vi "Forebrain Draw Buoy.vi"() -> ()   [LabVIEW 2012]
doc: "This VI contrains the Forebrain within the Olin Robot Architecture. It must be run first to load the appropriate mission definition files. It contains a finite state machine built around a tabbed Operator interface that will guide an operator through the startup, run shutdown mission sequence. After running it, run the Midbrain and Hindbrain VIS."
panel:
  in  "# 5":u8 max=5 step=1
  in  "# 4":u8 max=5 step=1
  in  "# 3":u8 max=5 step=1
  in  "# 2":u8 max=5 step=1
  in  "# 1":u8 max=5 step=1
  in  "# 0":u8 max=5 step=1
  in  "IR Servo":u8(knob)=7 scale=0.0..14.0
  out "return count":u32
  out "error out":errorcluster
  in  "error in 2":errorcluster
  out "Desired \nVelocity":i16=5
  out "Local\nHeading":i16=90
  out "Ycurrent":dbl format="%#_3g"
  out "Xcurrent":dbl format="%#_3g"
  out "Ystart":dbl
  out "Xstart":dbl
  in  "error in":errorcluster
  out "Robot Live":bool
  in  "E-Stop":bool
  in  "Tab":T1(tab)
  out "MissionTime (Min)":dbl(knob) scale=0.0..10.0
  out "LidarDist":i16
  out "IR Index":i32
  out "BatteryLevel":dbl(slide) scale=6.0..9.0
  out "String Received":string
  out "Send String":string="$B^"
  in  "VISA resource name":refnum<visa-resource-name>="COM10"
  in  "Mode":i16 min=0 max=99 step=1
  in  "Desired Vel":i16(slide) scale=-9.0..9.0
  in  "Local Head":i16(slide) scale=-180.0..180.0
  out "StartMissionMap":picture
  out "MapDARCheck":picture
  in  "RunRobot":bool
  in  "Tug letter":string="G"
  out "Tug X":i32
  out "Tug Y":i32
  out "Tug H":i32
  out "BS Time Out?":bool
  out "Buoy locations":cluster{"regular expression":string, i32, i32}[](array[cluster])
  out "Valid ?":bool
  out "Battery\nVolts":i16
  out "Base Station data rec'd":string
  out "udp rate":bool
  out "CollisionWarning":bool
  out "DebugMapDAR":picture
  in  "MapDAR Control":T2={"NumberOfBeams"=180, "SensorRange"=500.0, "Noise (0.1 to 1)"=0.0} {"Noise (0.1 to 1)" min=0.0 max=1.0 step=0.1; "SensorRange" min=500.0 max=1500.0 step=100.0; "NumberOfBeams" min=36 max=360 step=2}
  out "MapDAR Data (r:pixel b:degrees)":cluster{"Range":dbl, "Bearing":dbl}[](array[cluster])
  in  "Stop DebugSENSE":bool
  out "MissionMap":picture
  out "Tug position":T3
  out "initialized MDF":T4(array[cluster])
  out "Way Point Index":i32
  out "InitialWaypoint":cluster{"X":i16, "Y":i16}
  in  "Pen Color":u32(colorbox)=15671808
  in  "Select Pen Attributes":T5={"Width"=1, "Style"=enum."Solid"}
  out "Draw??":bool
  in  "WhereAmI?FromBase":T6
  out "(xr,yr)":cluster{"X":dbl, "Y":dbl}
  in  "RobotPosition":T3 {"xrobot" min=0.0 max=1177.0 step=10.0; "yrobot" min=0.0 max=850.0 step=10.0; "heading" min=0.0 max=7.0 step=0.1}
  out "MDF_Original":T4(array[cluster])
  out "WhatAroundMeMap?":cluster{"T":dbl, "Range":dbl, "Bearing":dbl}[](array[cluster])
  out "WayPointAct":dbl[](array[numeric])
  out "SteerAngle":dbl
  out "MissionDefFile":picture
  out "MDF":T4(array[cluster])
  in  "Select Your Behavior":T7(ring)
  out "No. of Waypoints":i32
  in  "Exit Planning":bool
  in  "BoatSpeed for Leg":dbl(slide) min=-9.0 max=9.0 step=1.0 scale=-9.0..9.0
  out "BuildMDF":bool
  out "WayPoint Position":cluster{"X":i32, "Y":i32}
  out "Send String to NXT":string="$B^"
  in  "Behavior Command":T7(ring)
  out "CollisionLight":bool
  out "Where? Manual":T6
  out "ActManual":bool
  in  "Manual Heading":i16(knob) min=-179 max=180 step=5 scale=180.0..-180.0
  out "MWhat?":bool
  out "Where? 2":bool
  out "How? 2":bool
  in  "ManualModeStop":bool
  out "ManualModeMapDAR":picture
  out "ManualMissionMap":picture
  out "Battery":dbl(slide) scale=0.0..8.0
  in  "Manual Vel":dbl(slide) min=-6.0 max=6.0 step=1.0 scale=-6.0..6.0
  out "MissionTime":dbl(knob) scale=0.0..10.0
  out "Heading":cluster{dbl, dbl}(knob)={0.0, 34.390870865624734} scale=180.0..-179.0 scale format="%#_3g"
  out "Speed":i16(knob) scale=-6.0..6.0
  out "Current Behavior":T7(ring)
  out "Robot Position":cluster{"X":dbl, "Y":dbl} {"X" format="%#_3g"; "Y" format="%#_3g"}
  out "Ready":bool
  in  "Pause":bool
  in  "Rerun MDF":bool
  out "CollisionLight 2":bool
  out "Act":bool
  out "Neo-C":bool
  out "How?":bool
  out "What?":bool
  out "A Heading":cluster{dbl, dbl}(knob)={0.0, 34.390870865624734} scale=180.0..-180.0
  out "A Speed":dbl(knob) scale=-9.0..9.0
  out "AutoBattery":dbl(slide) scale=0.0..8.0
  out "AutoModeLIDAR":picture
  out "AutoMissionMap":picture
  in  "RunAutoMode":bool
  out "MissionTimeAuto":dbl(knob) scale=0.0..60.0
  out "Where?":bool
  # "To run\nrobot,\nclick\narrow\nabove\n\nRun Robot button must be on"
  # "Operation Directions\n\n1)Click on Startup&\nShutdown tab.\n2) Click on Run \nArrow on menubar.\nRun Forebrain,\nvis from the project\nexplorer.\n3) Select a mssion \nmap file when asked.\n4) Check robot is \nfully operational on\nStartup tab.\n5) Debug with debug\ntabs as required.\n6) Select ManualMode\ntab and test drive \nrobot.\n7) Select PlanMission\ntab and set up \nmission.\n8) Go to AutoMode\ntab and run mission."
  # "Turns off drive\nmotors"
  # "Enter Olin Test  Pool"
  # "Xbee Com Port"
  # "xBee\"Send String\" (mode, desired velocity, local heading)"
  # "(Type in Tug Letter  L T G P  (look at boat cradle)"
  # "Should be on to\nrun"
  # "BoatG,X,Y,H,BoatT,X,Y,H,BoatP,X,Y.H,BoatL,X,Y,H,BuoyA,X,Y,BuoyB,X,Y,BuoyC,X,Y,BuoyD,X,Y,Time(hours,Min,Sec)"
  # "To stop  program \nturn off here"
  # "Use this tab\nto explore\nLIDAR\ndata and \noperation"
  # "Set\nNumberOfBeams\nSensorRange\nNoise\nto\nview\nsimulated\nsensor\ndata"
  # "Turn Debug Sim \nto leave this\ntab--->"
  # "This tab will auto\nreturn to Startup \nin 2 seconds"
  # "Clean up interface and make more useful for debugging behaviors"
  # "Build out interface and make more useful for debugging act"
  # "This tab will auto\nreturn to Startup \nin 2 seconds"
  # "Directions:\n1) Select Robot Behavior for each mission leg.\n2) Select Robot Speed for leg.\n3) Click on robots current location for first waypoint.\n4) Hold down button and drag to next\nwaypoint. Click on next leg waypoint.\n5) Hold mouse button down and drag to \nnext waypoint. \n6) Click on next waypoint. Repeat for full mission.\n7) MDF will store up to 20 waypoints."
  # "Remember to\nset boat\nleg speed !"
  # "Please Adjust Scroll Barrs in Tug Off Mode to Prevent  Extra Lines Being Drawn"
  # "\"Send String\" (mode, desired velocity, local heading)"
  # "Press to stop and return to StartUp"
  # "Open MidBrain\nArbiter to see\nBrain Waves"
  # "AutoMode\nAutomatically \nReturns to \nStartUp Mode"
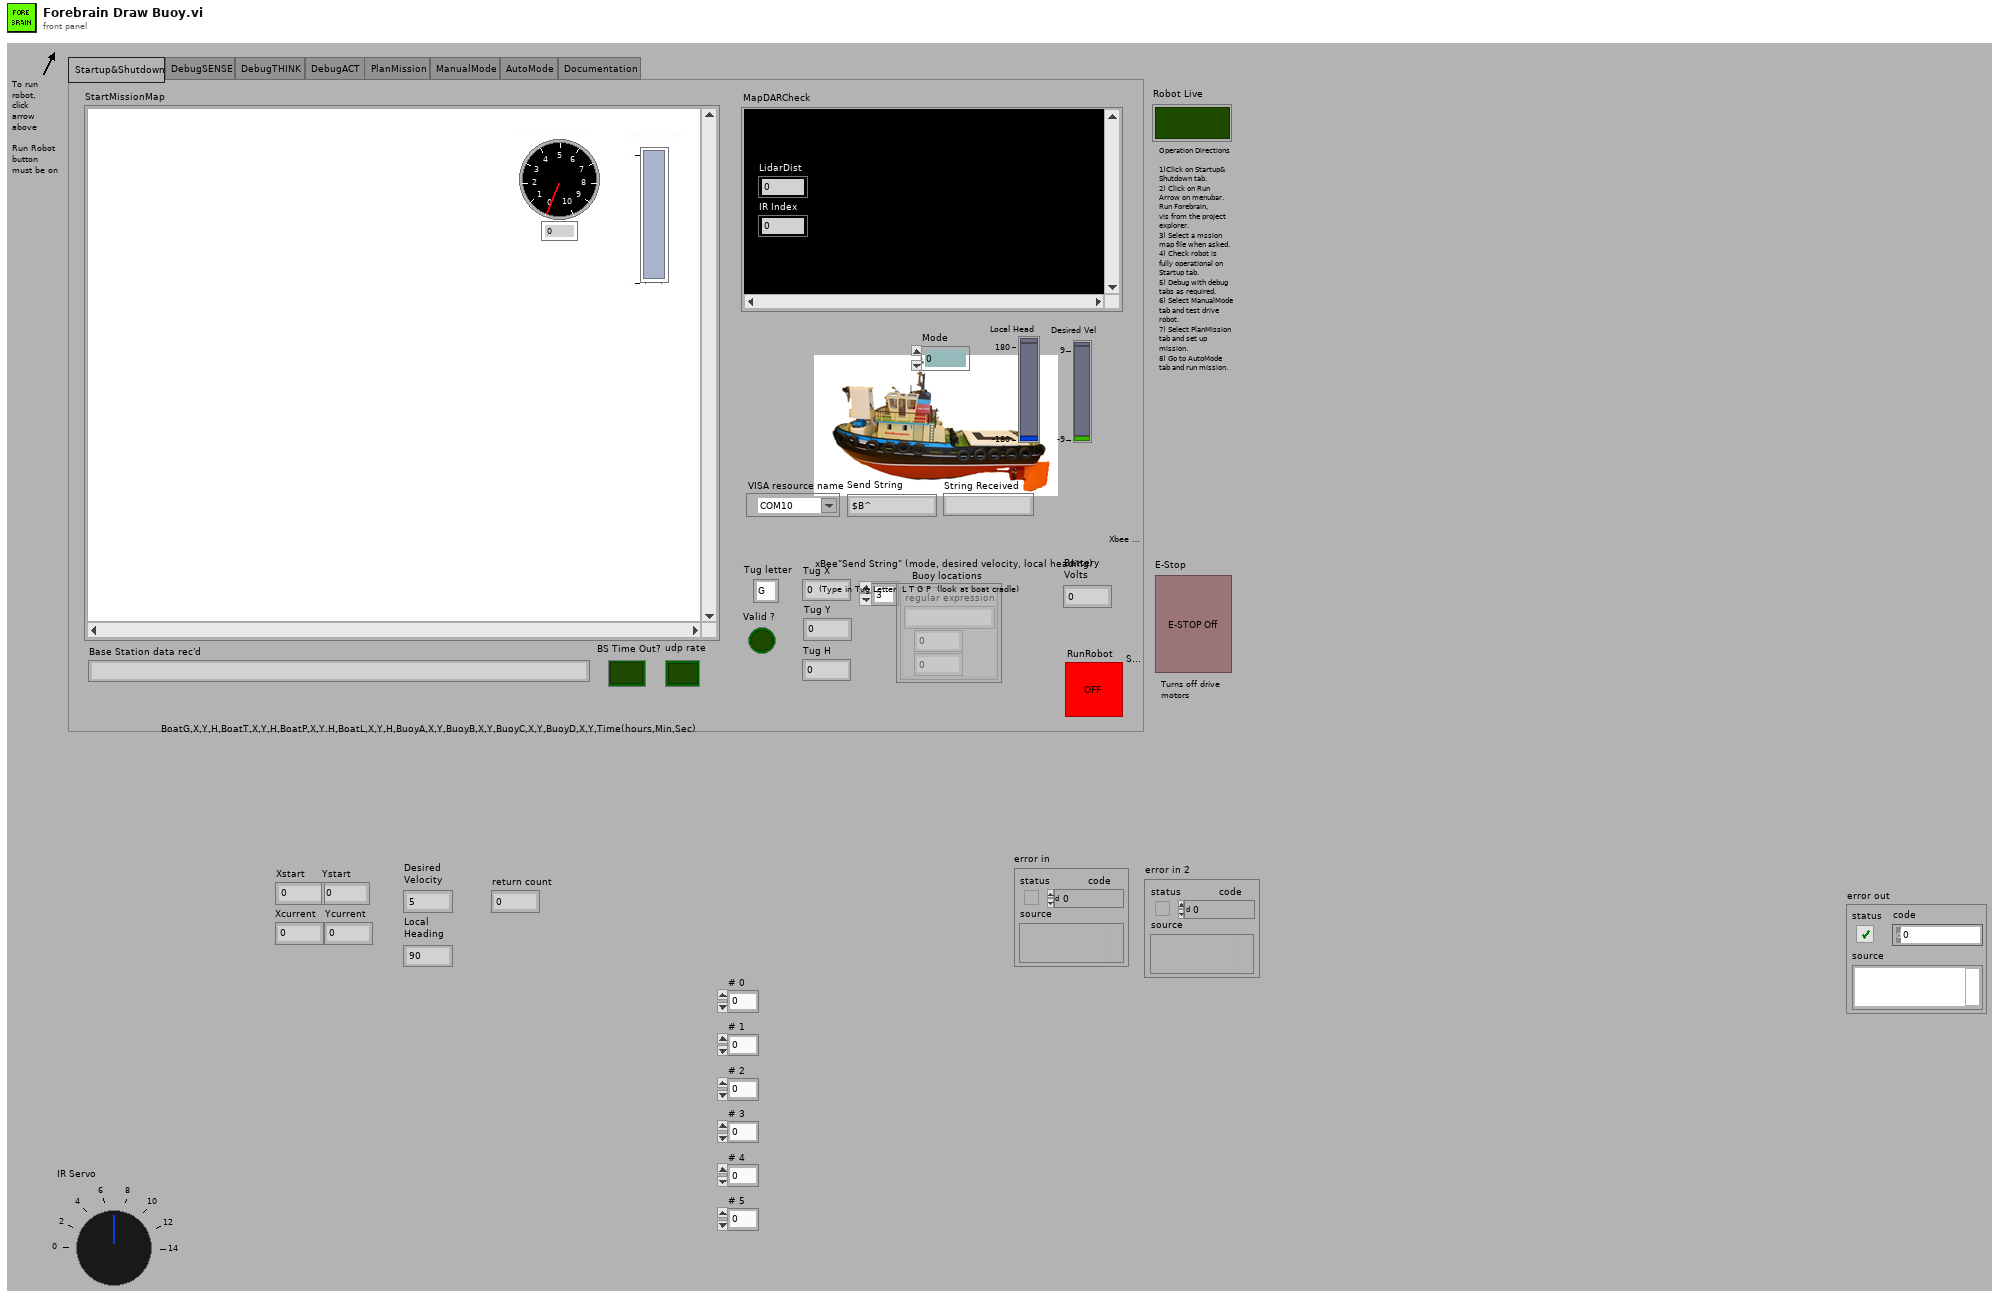
[diagram p1: front panel]
types:
  T1 = enum32{"Startup&Shutdown", "DebugSENSE", "DebugTHINK", "DebugACT", "PlanMission", "ManualMode", "AutoMode", "Documentation"}
  T2 = cluster{"NumberOfBeams":i32, "SensorRange":dbl, "Noise (0.1 to 1)":dbl}
  T3 = cluster{"xrobot":dbl, "yrobot":dbl, "heading":dbl}
  T4 = cluster{"Status":enum16{"Past", "Current", "Future"}, "x":dbl, "y":dbl, "z":dbl, "Vel":dbl, "Dwell Time":dbl, "BehCom":enum16{"Tug Off", "Manual Mode", "Goto WayPoint", "Back Up", "Circle", "Left Wall Follow", "Right Wall Follow", "Hunt"}, "Expand1":dbl, "Expand2":dbl, "Expand3":dbl}[]
  T5 = cluster{"Width":u16, "Style":enum32{"Solid", "Dash", "Dot", "DashDot", "DashDotDot"}}
  T6 = cluster{"T":dbl, "X":dbl, "Y":dbl, "Direction":dbl}
  T7 = enum16{"Tug Off", "Manual Mode", "Goto WayPoint", "Back Up", "Circle", "Left Wall Follow", "Right Wall Follow", "Hunt"}
  T8 = cluster{"VelCom":dbl, "BehCom":enum16{"OpenFieldTransit", "P-WallFollow", "S-WallFollow", "LaneFollow", "ManualMode"}}
  T9 = typedef "IMAQ Image.ctl" = refnum<image>
  T10 = typedef "imagedata.ctl" = cluster{"image type":i32, "image depth":i32, "image":u8[], "mask":u8[], "colors":u32[], "Rectangle":cluster{"left":i16, "top":i16, "right":i16, "bottom":i16}}
  T11 = cluster{"Status":enum16{"Past", "Current", "Future"}, "x":dbl, "y":dbl, "z":dbl, "Vel":dbl, "Dwell Time":dbl, "BehCom":enum16{"Tug Off", "Manual Mode", "Goto WayPoint", "Back Up", "Circle", "Left Wall Follow", "Right Wall Follow", "Hunt"}, "Expand1":dbl, "Expand2":dbl, "Expand3":dbl}
  T12 = typedef "LVMouseTypeDef.ctl" = cluster{"Mouse Position":cluster{"X":i32, "Y":i32}, "Mouse Modifiers":cluster{"Button Down":bool, "Shift Mod":bool, "Menu Mod":bool, "Option Mod":bool}}
  T13 = cluster{"regular expression":string, i32, i32, i32}
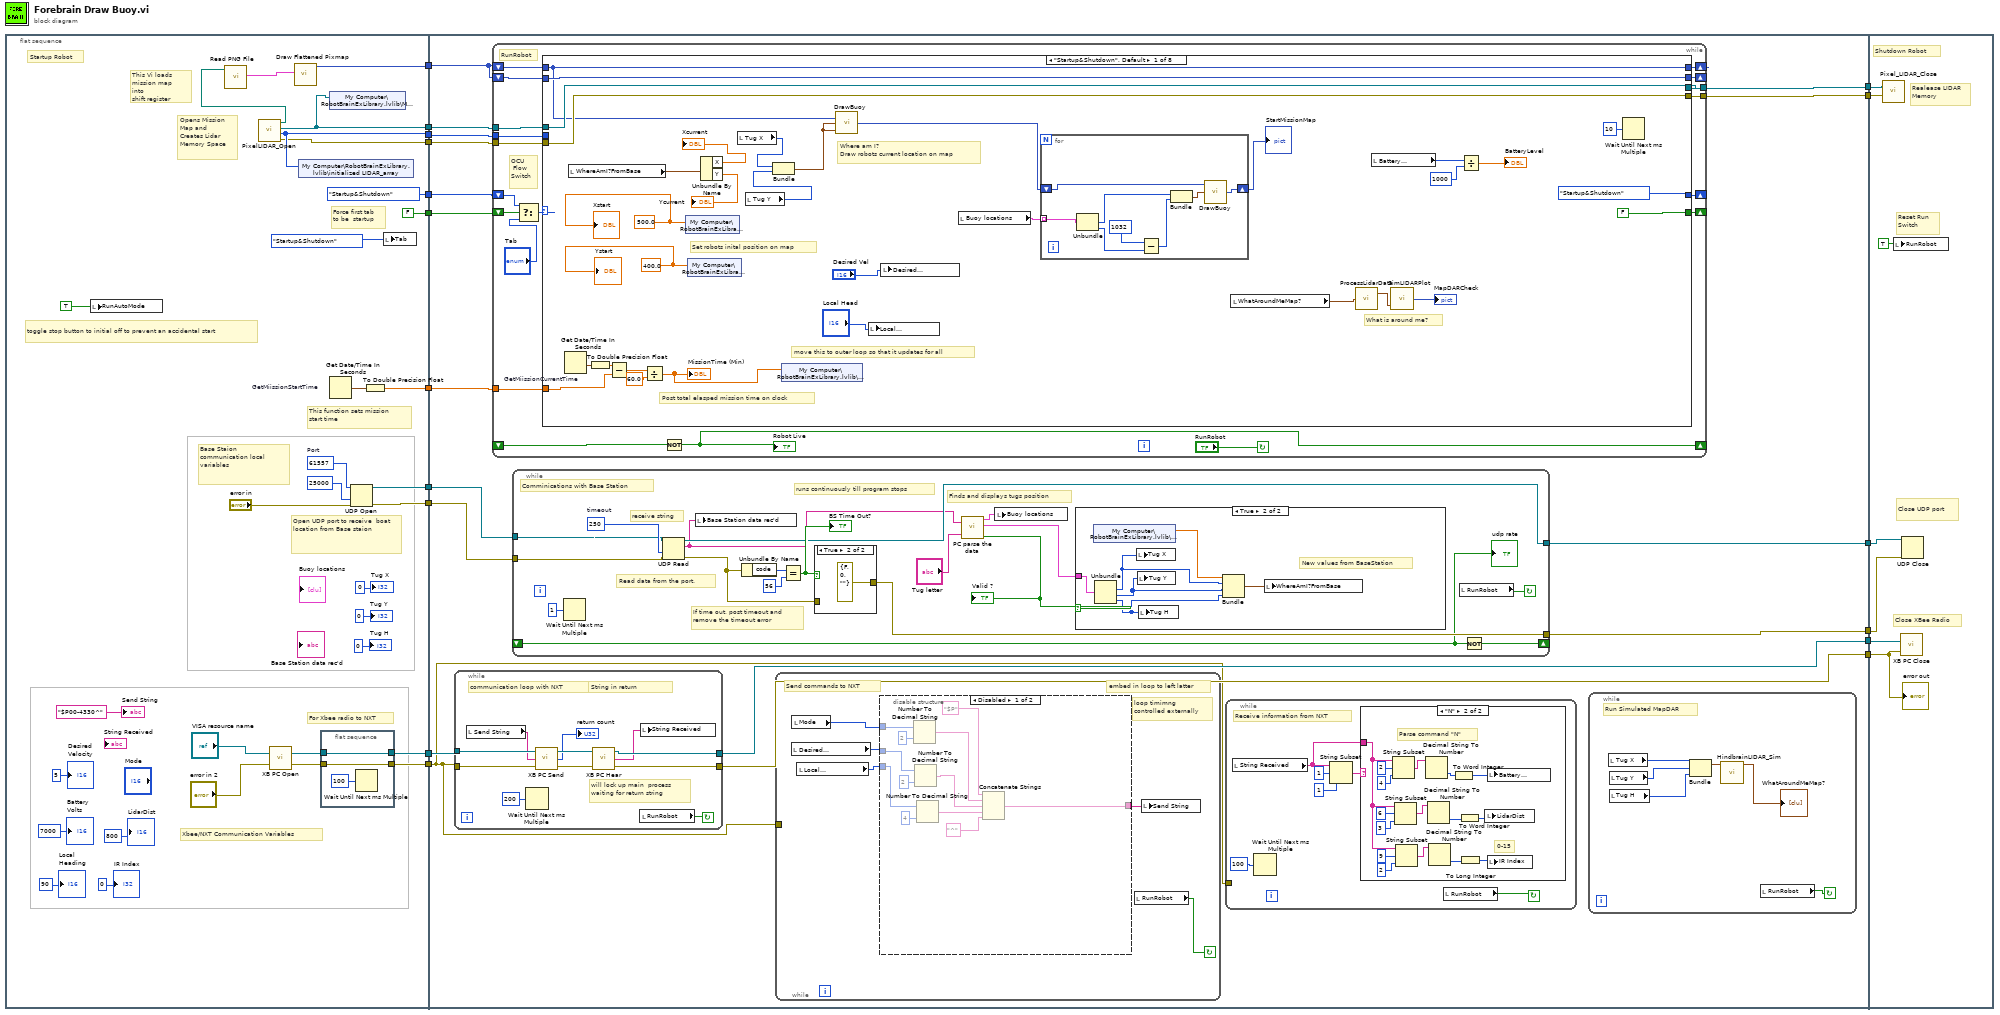
[diagram p0: block diagram]
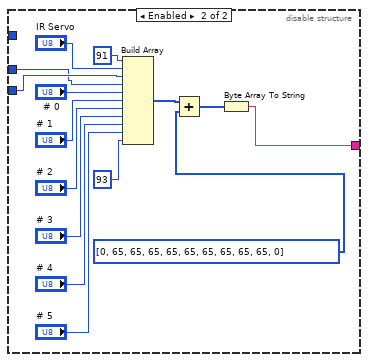
[diagram p5: hidden frame]
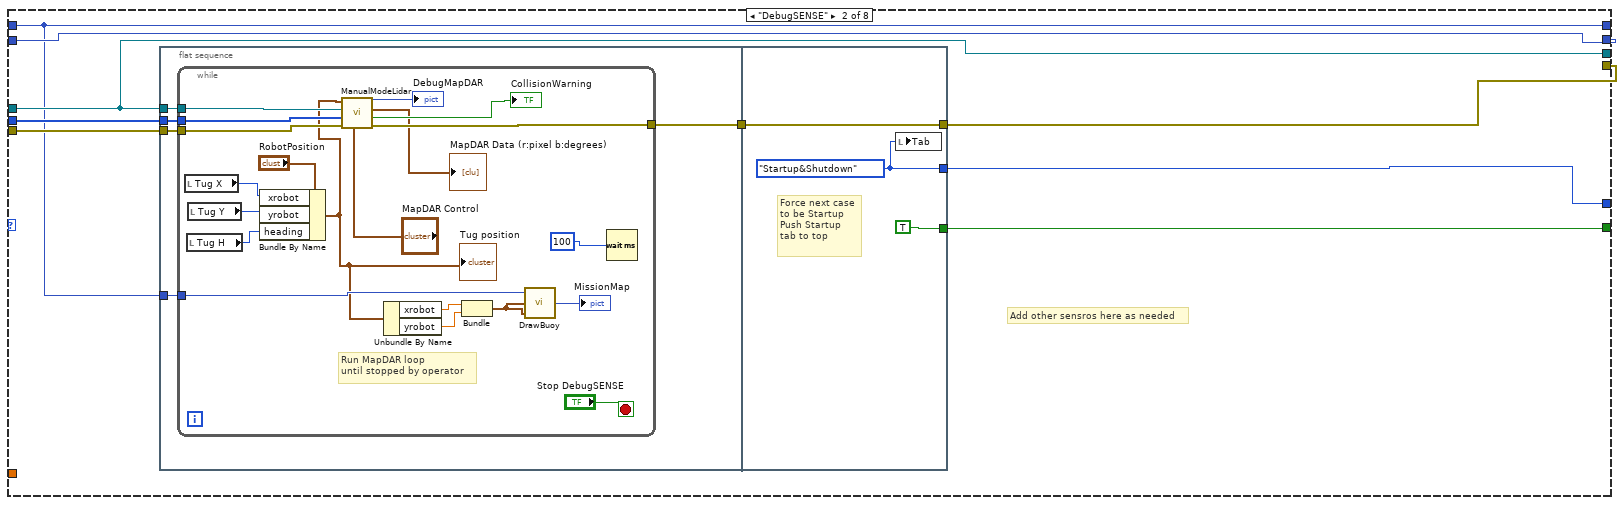
[diagram p6: hidden frame]
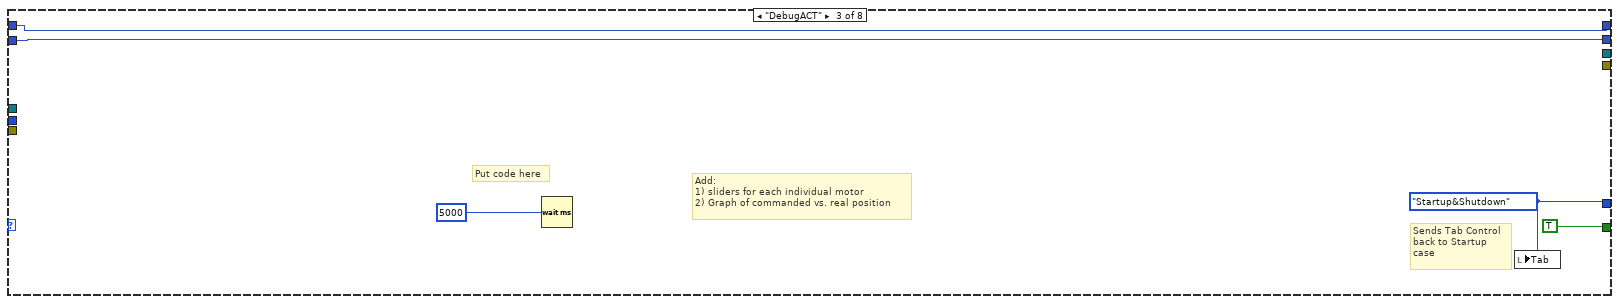
[diagram p7: hidden frame]
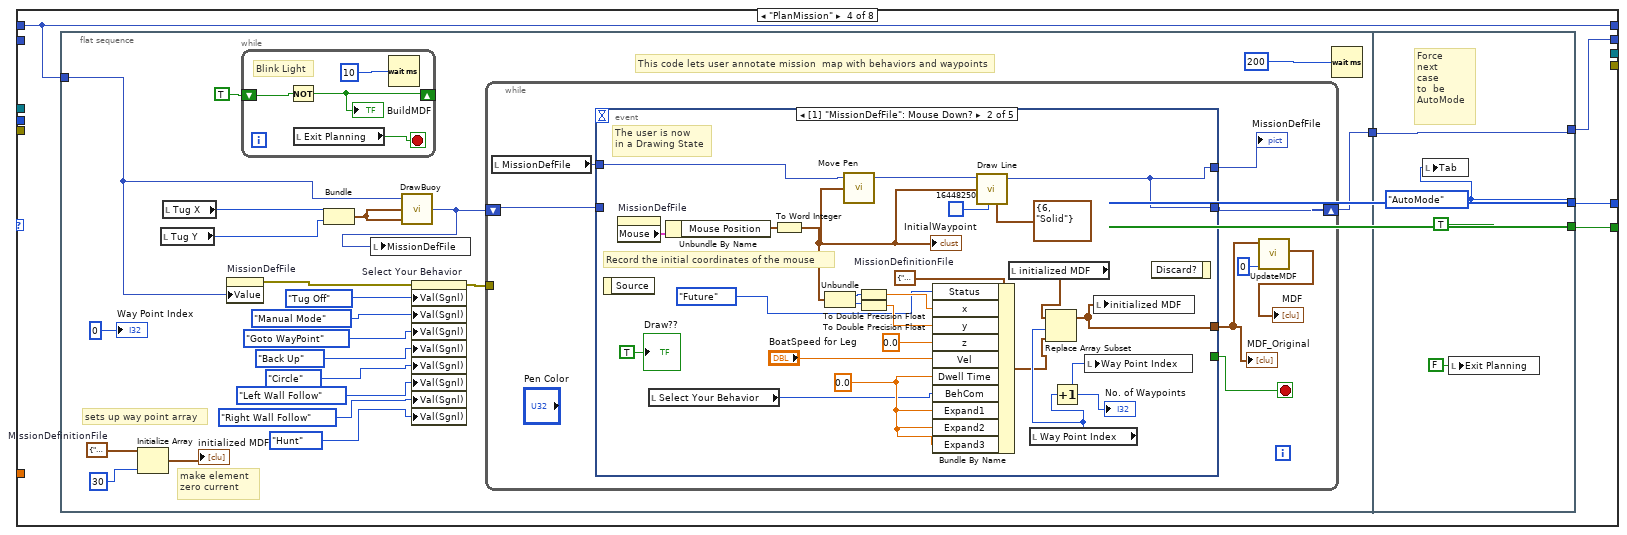
[diagram p8: hidden frame]
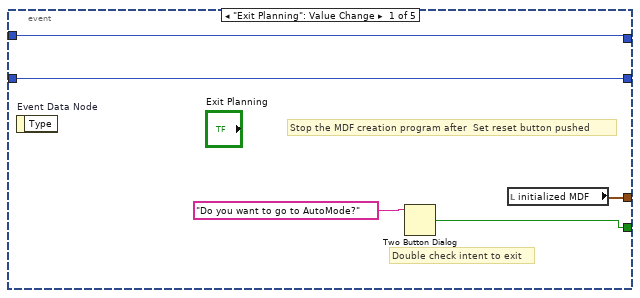
[diagram p9: hidden frame]
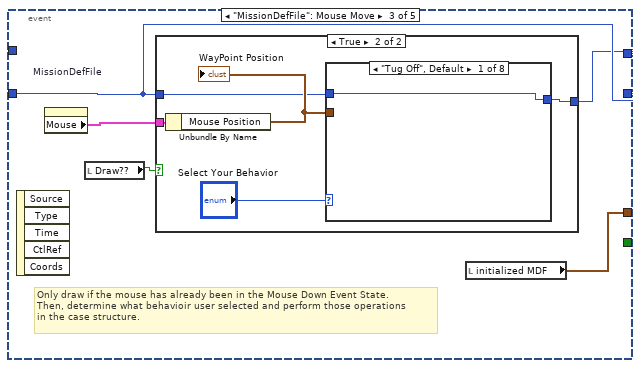
[diagram p10: hidden frame]
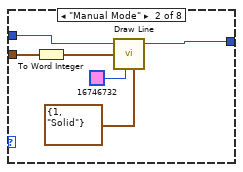
[diagram p12: hidden frame]
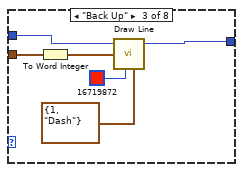
[diagram p13: hidden frame]
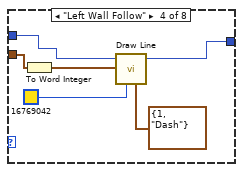
[diagram p14: hidden frame]
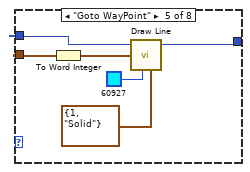
[diagram p15: hidden frame]
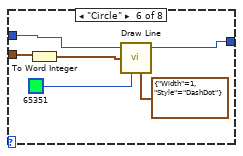
[diagram p16: hidden frame]
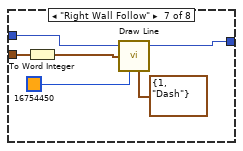
[diagram p17: hidden frame]
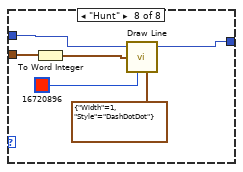
[diagram p18: hidden frame]
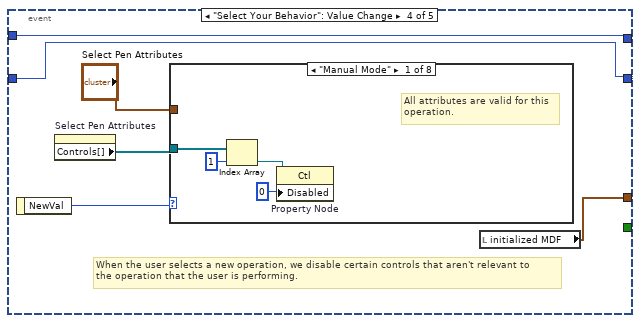
[diagram p19: hidden frame]
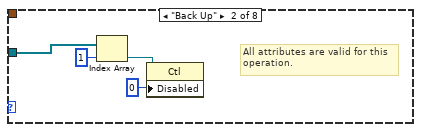
[diagram p20: hidden frame]
diagram:
  n1 = flat-sequence {
    tunnel: [w48] -> w17
    tunnel: [w47] -> w16
    tunnel: [w44] -> w15
    tunnel: [w46] -> w14
    tunnel: [w45] -> w13
    tunnel: [FALSE ("RunAutoMode")] -> w10
    tunnel: [T1."Startup&Shutdown" ("Tab")] -> w9
    tunnel: [w31] -> w8
    tunnel: [w30] -> w7
    tunnel: [w19] -> w6
    tunnel: [w18] -> w5
    tunnel: w17 -> [w69]
    tunnel: w16 -> [w68]
    tunnel: w15 -> [w67]
    tunnel: w14 -> [w66]
    tunnel: w13 -> [w65]
    tunnel: [w64] -> w12
    tunnel: [w63] -> w11
    tunnel: w10 -> [w62]
    tunnel: w9 -> [w61]
    tunnel: w8 -> [w56]
    tunnel: w7 -> [w55]
    tunnel: w6 -> [w60]
    tunnel: w5 -> [w57]
    tunnel: [w59] -> w4
    tunnel: [w58] -> w3
    tunnel: [w54] -> w2
    tunnel: [w53] -> w1
    tunnel: w12 -> [w615]
    tunnel: w11 -> [w614]
    tunnel: w4 -> [w613]
    tunnel: w3 -> [w612]
    tunnel: w2 -> [w611]
    tunnel: w1 -> [w610]
    frame #0 {
      w37 = u16 61557  # Port
      # "For Xbee radio to NXT"
      # "Xbee/NXT Communication Variables"
      # "Base Staion communication local variables"
      # "Open UDP port to receive  boat location from Base staion"
      # "Force first tab\nto be  startup"
      # "toggle stop button to initial off to prevent an accidental start"
      # "Opens Mission\nMap and\nCreates Lidar\nMemory Space"
      # "This function sets mission \nstart time"
      # "This Vi loads\nmission map into \nshift register"
      # "Startup Robot"
      n2 = local write "RunAutoMode"(TRUE ("RunAutoMode")) -> ()
      n3 = call "PixelLIDAR_Open.vi"() -> ("error out"=w45:errorcluster, "initialized LIDAR\narray"=w46:i32[], "MDF Image"=w44:T9, "MissionMap"=w39:path)  [unwired: 2 in]
      n4 = call <vilib>:"Read PNG File.vi"("path to PNG file"=w39) -> ("image data"=w38:T10)  [unwired: 8 in, 2 out]
      n5 = call "XB PC Open.vi"("error in (no error)"="error in 2", "VISA resource name"="VISA resource name") -> ("error out"=w22:errorcluster, "VISA resource name out"=w23:refnum<visa-resource-name>)
      n6 = call <vilib>:"Draw Flattened Pixmap.vi"("image data"=w38) -> ("new picture"=w47:picture)  [unwired: 8 in]
      n7 = shared-variable "My Computer\\RobotBrainExLibrary.lvlib\\initialized LIDAR_array"(w46) -> ()  [unwired: 1 in, 1 out]
      n8 = flat-sequence {
        tunnel: w23 -> [w50]
        tunnel: w22 -> [w51]
        tunnel: [w51] -> w18
        tunnel: [w50] -> w19
        frame #0 {
          n9 = Wait Until Next ms Multiple(millisecond multiple=u32 100) -> ()  [unwired: 1 out]
        }
      }
      n10 = shared-variable "My Computer\\RobotBrainExLibrary.lvlib\\MDF Image"(w44) -> ()  [unwired: 1 in, 1 out]
      n11 = Get Date/Time In Seconds "GetMiissionStartTime"() -> (seconds since 1Jan1904=w49:timestamp)
      n12 = UDP Open(8:"error in", 9:25000 ("timeout ms (25000)"), 11:w37) -> (port=w31:refnum<k16>, 0:w30:errorcluster)  [unwired: 2 in, 1 out]
      n13 = To Double Precision Float(number=w49) -> (double precision float=w48:dbl)
      n14 = local write "Tab"(T1."Startup&Shutdown" ("Tab")) -> ()
      "Tug X" <- 0 ("Tug X")
      "Tug Y" <- 0 ("Tug Y")
      "Tug H" <- 0 ("Tug H")
      "Battery\nVolts" <- i16 7000 ("Battery\nVolts")
      "LidarDist" <- i16 800 ("Dist")
      "IR Index" <- 0 ("IR Index")
      "Local\nHeading" <- i16 90 ("Local\nHeading")
      "Desired \nVelocity" <- i16 5 ("Desired \nVelocity")
      "Send String" <- "$P00-4330^"
    }
    frame #1 {
      n15 = while {
        tunnel: w60 -> [w166]
        tunnel: w57 -> [w165]
        tunnel: [w162] -> w58
        tunnel: [w161] -> w59
        stop <- w160 continue-if-true
        # "will lock up main  process\nwaiting for return string"
        # "communication loop with NXT"
        # "send a string to the NXT and receive a String in return"
        n16 = local read "Send String"() -> (w158:string)
        n17 = Wait Until Next ms Multiple(millisecond multiple=u32 200) -> ()  [unwired: 1 out]
        n18 = call "XB PC Send.vi"("error in (no error)"=w165, "String"=w158, "VISA resource name"=w166) -> ("error out"=w164:errorcluster, "return count"=→"return count":u32, "VISA resource name out"=w163:refnum<visa-resource-name>)
        n19 = call "XB PC Hear.vi"("VISA resource name"=w163, "error in (no error)"=w164) -> ("VISA resource name out"=w161:refnum<visa-resource-name>, "String Received"=w157:string, "error out"=w162:errorcluster)
        n20 = local read "RunRobot"() -> (w160:bool)
        n21 = local write "String Received"(w157) -> ()
      }
      n22 = while {
        shift-right: [w167] -> _
        shift-left: _ -> [w184]
        shift-right: [w183] -> _
        shift-left: w61 -> [w182]
        shift-right: [w179] -> _
        shift-left: w62 -> [w178]
        tunnel: w69 -> [w177]
        shift-right: [w175] -> _
        shift-left: w68 -> [w176]
        shift-right: [w173] -> _
        shift-left: w68 -> [w174]
        tunnel: w67 -> [w172]
        tunnel: w66 -> [w171]
        tunnel: w65 -> [w170]
        tunnel: [w169] -> w64
        tunnel: [w168] -> w63
        stop <- "RunRobot" continue-if-true
        # "RunRobot"
        # "OCU\n Flow\nSwitch"
        n23 = Select(t=w182, s=w178, f="Tab") -> (s? t:f=w180:T1)
        n24 = case shown="\"Startup&Shutdown\", Default" w180 {
          selector: w180 -> [_ _ _ _ _ w513 _ _]
          tunnel: [T1."Startup&Shutdown" ("Tab") w230 w265 w272 w439 w514 T1."Startup&Shutdown" ("Tab") w608] -> w183
          tunnel: [FALSE ("s") w229 TRUE ("s") w271 w440 w512 FALSE ("s") TRUE ("s")] -> w179
          tunnel: w177 -> [w211 _ _ _ w437 w510 _ _]
          tunnel: w176 -> [w204 w226 w264 w268 w435 w507 w601 w606]
          tunnel: [w204 w226 w264 w268 w435 w507 w601 w606] -> w175
          tunnel: w174 -> [w210 w227 w263 _ w436 w509 w600 w605]
          tunnel: [w210 w227 w263 w269 w436 w509 w600 w605] -> w173
          tunnel: w172 -> [w209 w228 _ _ _ _ _ _]
          tunnel: w171 -> [_ w234 _ _ _ _ _ _]
          tunnel: w170 -> [w208 w233 _ _ _ _ _ _]
          tunnel: [w209 w228 _ _ _ _ _ _] -> w169
          tunnel: [w208 w232 _ _ _ _ _ _] -> w168
          frame "Startup&Shutdown", Default {
            w199 = 400.0 ("Ystart")
            w200 = 500.0 ("Xstart")
            # "move this to outer loop so that it updates for all"
            # "Where am I?\nDraw robots current location on map"
            # "Post total elasped mission time on clock"
            # "What is around me?"
            # "Set robots inital position on map"
            n25 = Get Date/Time In Seconds "GetMiissionCurrentTime"() -> (seconds since 1Jan1904=w215:timestamp)
            n26 = local read "WhereAmI?FromBase"() -> (w189:T6)
            n27 = To Double Precision Float(number=w215) -> (double precision float=w214:dbl)
            n28 = Subtract(x=w214, y=w211) -> (x-y=w213:dbl)
            n29 = Divide(x=w213, y=60.0) -> (x/y=w207:dbl)
            "MissionTime (Min)" <- w207
            n30 = shared-variable "My Computer\\RobotBrainExLibrary.lvlib\\Xstart"(w200) -> ()  [unwired: 1 in, 1 out]
            n31 = shared-variable "My Computer\\RobotBrainExLibrary.lvlib\\Ystart"(w199) -> ()  [unwired: 1 in, 1 out]
            n32 = Unbundle By Name(w189) -> ("X"=→"Xcurrent":dbl, "Y"=→"Ycurrent":dbl)
            n33 = local read "Tug X"() -> (w198:i32)
            n34 = local read "Tug Y"() -> (w197:i32)
            n35 = Bundle("Tug X"=w198, "Tug Y"=w197) -> (w203:cluster{"Tug X":i32, "Tug Y":i32})  [unwired: 1 in]
            n36 = shared-variable "My Computer\\RobotBrainExLibrary.lvlib\\MissionTime"(w207) -> ()  [unwired: 1 in, 1 out]
            n37 = call "DrawBuoy.vi"("(xr,yr) old"=w203, "(xr,yr) new"=w203, "2D Picture"=w204) -> ("new picture"=w187:picture)
            n38 = local write "Local\nHeading"("Local Head") -> ()
            n39 = local write "Desired \nVelocity"("Desired Vel") -> ()
            n40 = local read "Buoy locations"() -> (w188:cluster{"regular expression":string, i32, i32}[])
            n41 = for {
              tunnel: w188 -> [w223] mode=indexing
              shift-right: [w224] -> w186
              shift-left: w187 -> [w225]
              n42 = Unbundle(w223) -> (w219:i32, w222:i32)  [unwired: 1 out]
              n43 = Subtract(x=1032, y=w222) -> (x-y=w221:i32)
              n44 = Bundle(w219, w221) -> (w218:cluster{i32, i32})  [unwired: 1 in]
              n45 = call "DrawBuoy.vi"("(xr,yr) new"=w218, "2D Picture"=w225) -> ("new picture"=w224:picture)  [unwired: 1 in]
            }
            "StartMissionMap" <- w186
            n46 = local read "WhatAroundMeMap?"() -> (w190:cluster{"T":dbl, "Range":dbl, "Bearing":dbl}[])
            n47 = call "ProcessLidarData.vi"("WhatAroundMe?MM"=w190) -> ("data array [mag, phase (deg)]"=w205:cluster{"magnitude":dbl, "phase":dbl}[])  [unwired: 1 out]
            n48 = local read "Battery\nVolts"() -> (w194:i16)
            n49 = call "SimLIDARPlot.vi"("data array [mag, phase (deg)]"=w205) -> ("SONAR"=→"MapDARCheck":picture)  [unwired: 1 in]
            n50 = Divide(x=w194, y=i16 1000) -> (x/y=→"BatteryLevel":dbl)
            n51 = Wait Until Next ms Multiple(millisecond multiple=u32 10) -> ()  [unwired: 1 out]
            "Xstart" <- w200
            "Ystart" <- w199
          }
          frame "DebugSENSE" {
            # "Add other sensros here as needed"
            n52 = flat-sequence {
              tunnel: w234 -> [w239]
              tunnel: w233 -> [w238]
              tunnel: w228 -> [w237]
              tunnel: [w236] -> w231
              tunnel: w226 -> [w235]
              tunnel: [w262] -> w232
              tunnel: w231 -> [w262]
              tunnel: [w261] -> w230
              tunnel: [TRUE ("s")] -> w229
              frame #0 {
                n53 = while {
                  tunnel: w239 -> [w259]
                  tunnel: w238 -> [w258]
                  tunnel: w237 -> [w257]
                  tunnel: [w256] -> w236
                  tunnel: w235 -> [w250]
                  stop <- "Stop DebugSENSE" stop-if-true
                  # "Run MapDAR loop\nuntil stopped by operator"
                  n54 = local read "Tug X"() -> (w244:i32)
                  n55 = local read "Tug H"() -> (w245:i32)
                  n56 = local read "Tug Y"() -> (w243:i32)
                  n57 = Bundle By Name(cluster="RobotPosition", "xrobot"=w244, "yrobot"=w243, "heading"=w245) -> (w241:T3)
                  "Tug position" <- w241
                  n58 = call "ManualModeLidar.vi"("LIDARControl"="MapDAR Control", "error in"=w258, "initialized \nsonar ray\narray"=w259, "MDF Image"=w257, "SubPosition"=w241) -> ("error out"=w256:errorcluster, "Collision\nWarning"=→"CollisionWarning":bool, "LIDAR Data (r:pixel b:degrees)"=→"MapDAR Data (r:pixel b:degrees)":cluster{"Range":dbl, "Bearing":dbl}[], "LIDAR"=→"DebugMapDAR":picture)  [unwired: 1 in]
                  n59 = Unbundle By Name(w241) -> ("xrobot"=w248:dbl, "yrobot"=w247:dbl)
                  n60 = Bundle("xrobot"=w248, "yrobot"=w247) -> (w240:cluster{"xrobot":dbl, "yrobot":dbl})  [unwired: 1 in]
                  n61 = call "DrawBuoy.vi"("(xr,yr) old"=w240, "(xr,yr) new"=w240, "2D Picture"=w250) -> ("new picture"=→"MissionMap":picture)
                  n62 = Wait (ms)(milliseconds to wait=u32 100) -> ()  [unwired: 1 out]
                }
              }
              frame #1 {
                w261 = T1."Startup&Shutdown" ("Tab")
                # "Force next case\nto be Startup\nPush Startup\ntab to top"
                n63 = local write "Tab"(w261) -> ()
              }
            }
          }
          frame "DebugACT" {
            w265 = T1."Startup&Shutdown" ("Tab")
            # "Add:\n1) sliders for each individual motor\n2) Graph of commanded vs. real position"
            # "Put code here"
            # "Sends Tab Control\nback to Startup\ncase"
            n64 = Wait (ms)(milliseconds to wait=u32 5000) -> ()  [unwired: 1 out]
            n65 = local write "Tab"(w265) -> ()
          }
          frame "PlanMission" {
            n66 = flat-sequence {
              tunnel: [w293] -> w270
              tunnel: w268 -> [w286]
              tunnel: [w433] -> w272
              tunnel: [TRUE ("s")] -> w271
              tunnel: w270 -> [w432]
              tunnel: [w432] -> w269
              frame #0 {
                w284 = T11 {"Status"=enum."Future", "x"=0.0, "y"=0.0, "z"=0.0, "Vel"=0.0, "Dwell Time"=0.0, "BehCom"=enum."Tug Off", "Expand1"=0.0, "Expand2"=0.0, "Expand3"=0.0}  # MissionDefinitionFile
                # "make element \nzero current"
                # "sets up way point array"
                # "This code lets user annotate mission  map with behaviors and waypoints"
                n67 = Initialize Array ("Initialize WaypointArray")(w284, 30 ("dimension size")) -> (→"initialized MDF":T4)
                n68 = local read "Tug Y"() -> (w281:i32)
                n69 = local read "Tug X"() -> (w282:i32)
                n70 = property on="MissionDefFile" class="Pict"("Value"=w286) -> (error out=w291:errorcluster)  [unwired: 2 in, 1 out]
                n71 = while {
                  shift-right: [w297] -> _
                  shift-left: TRUE -> [w298]
                  stop <- w296 stop-if-true
                  # "Blink Light"
                  n72 = Not(x=w298) -> (.not. x?=w297:bool)
                  "BuildMDF" <- w297
                  n73 = local read "Exit Planning"() -> (w296:bool)
                  n74 = Wait (ms)(milliseconds to wait=u32 10) -> ()  [unwired: 1 out]
                }
                n75 = Bundle("Tug X"=w282, "Tug Y"=w281) -> (w287:cluster{"Tug X":i32, "Tug Y":i32})  [unwired: 1 in]
                n76 = call "DrawBuoy.vi"("(xr,yr) old"=w287, "(xr,yr) new"=w287, "2D Picture"=w286) -> ("new picture"=w285:picture)
                n77 = local write "MissionDefFile"(w285) -> ()
                n78 = property on="Select Your Behavior" class="Enum (strict)"(error in=w291, "Val(Sgnl)"=T7."Tug Off" ("Value (Signaling)"), "Val(Sgnl)"=T7."Manual Mode" ("Value (Signaling)"), "Val(Sgnl)"=T7."Goto WayPoint" ("Value (Signaling)"), "Val(Sgnl)"=T7."Back Up" ("Value (Signaling)"), "Val(Sgnl)"=T7."Circle" ("Value (Signaling)"), "Val(Sgnl)"=T7."Left Wall Follow" ("Value (Signaling)"), "Val(Sgnl)"=T7."Right Wall Follow" ("Value (Signaling)"), "Val(Sgnl)"=T7."Hunt" ("Value (Signaling)")) -> (error out=w292:errorcluster)  [unwired: 1 in, 1 out]
                n79 = while {
                  shift-right: [w305] -> w293
                  shift-left: w285 -> [w306]
                  tunnel: w292 -> [_]
                  stop <- w304 stop-if-true
                  n80 = local read "MissionDefFile"() -> (w303:picture)
                  n81 = event shown="[1] \"MissionDefFile\": Mouse Down?" {
                    selector: _ -> [_ _ _ _ _]
                    dyn-events: _ -> [_ _ _ _ _]
                    timeout: _ -> [_ _ _ _ _]
                    tunnel: [w309 w317 w337 w390 w428] -> w305
                    tunnel: w306 -> [w309 _ w337 w390 _]
                    tunnel: [w310 _ _ _ _] -> w304
                    tunnel: [w308 w332 w338 w392 w429] -> w300
                    tunnel: w303 -> [w307 w318 _ w391 w428]
                    tunnel: [w307 w317 w336 w391 w428] -> w302
                    event "Exit Planning": Value Change {
                      # "Double check intent to exit"
                      # "Stop the MDF creation program after  Set reset button pushed"
                      n82 = event-data "Event Data Node"() -> ()  [unwired: 1 in, 1 out]
                      n83 = Two Button Dialog(message="Do you want to go to AutoMode?") -> (T button?=w310:bool)  [unwired: 2 in]
                      n84 = local read "initialized MDF"() -> (w308:T4)
                    }
                    event "MissionDefFile": Mouse Down? {
                      w316 = T11 {"Status"=enum."Future", "x"=0.0, "y"=0.0, "z"=0.0, "Vel"=0.0, "Dwell Time"=0.0, "BehCom"=enum."Tug Off", "Expand1"=0.0, "Expand2"=0.0, "Expand3"=0.0}  # MissionDefinitionFile
                      w326 = 0.0 ("Dwell Time")
                      # "Record the initial coordinates of the mouse"
                      # "The user is now\nin a Drawing State"
                      n85 = event-data() -> ()  [unwired: 1 in, 1 out]
                      n86 = property on="MissionDefFile" class="Pict"() -> ("Mouse"=w335:T12)  [unwired: 2 in, 2 out]
                      n87 = local read "Select Your Behavior"() -> (w313:T7)
                      n88 = Unbundle By Name(w335) -> ("Mouse Position"=w333:cluster{"X":i32, "Y":i32})
                      n89 = To Word Integer(number=w333) -> (16bit integer=w321:cluster{"X":i16, "Y":i16})
                      "InitialWaypoint" <- w321
                      n90 = Unbundle(w321) -> ("X"=w330:i16, "Y"=w329:i16)
                      n91 = call <vilib>:"Move Pen.vi"("new position"=w321, "picture"=w318) -> ("new picture"=w322:picture)  [unwired: 3 in]
                      n92 = To Double Precision Float(number=w330) -> (double precision float=w328:dbl)
                      n93 = To Double Precision Float(number=w329) -> (double precision float=w327:dbl)
                      n94 = Bundle By Name(cluster=w316, "Status"=enum16{"Past", "Current", "Future"}."Future", "x"=w328, "y"=w327, "z"=0.0, "Vel"="BoatSpeed for Leg", "Dwell Time"=w326, "BehCom"=w313, "Expand1"=w326, "Expand2"=w326, "Expand3"=w326) -> (w312:T11)
                      n95 = call <vilib>:"Draw Line.vi"("picture"=w322, "end point"=w321, "color(black)"=u32 16448250, "pen"=T5 {"Width"=6, "Style"=enum."Solid"}) -> ("new picture"=w317:picture)  [unwired: 5 in]
                      n96 = local read "initialized MDF"() -> (w331:T4)
                      n97 = local read "Way Point Index"() -> (w314:i32)
                      n98 = Replace Array Subset(array=w331, new element=w312, index=w314) -> (w332:T4)
                      n99 = Increment(x=w314) -> (x+1=w334:i32)
                      "No. of Waypoints" <- w334
                      n100 = local write "Way Point Index"(w334) -> ()
                      n101 = local write "initialized MDF"(w332) -> ()
                      n102 = event-data() -> ()  [unwired: 2 in, 1 out]
                      "Draw??" <- TRUE ("Draw??")
                    }
                    event "MissionDefFile": Mouse Move {
                      # "Only draw if the mouse has already been in the Mouse Down Event State.\nThen, determine what behavioir user selected and perform those operations\nin the case structure."
                      n103 = event-data() -> ()  [unwired: 1 in, 5 out]
                      n104 = property on="MissionDefFile" class="Pict"() -> ("Mouse"=w340:T12)  [unwired: 2 in, 2 out]
                      n105 = local read "Draw??"() -> (w339:bool)
                      n106 = case shown="True" w339 {
                        tunnel: w340 -> [_ w346]
                        tunnel: w337 -> [w341 w342]
                        tunnel: [w341 w343] -> w336
                        frame False {
                        }
                        frame True {
                          n107 = Unbundle By Name(w346) -> ("Mouse Position"=w344:cluster{"X":i32, "Y":i32})
                          "WayPoint Position" <- w344
                          n108 = case shown="\"Tug Off\", Default" "Select Your Behavior" {
                            tunnel: w344 -> [_ w352 w358 w361 w367 w372 w378 w384]
                            tunnel: [w347 w353 w359 w363 w366 w373 w379 w385] -> w343
                            tunnel: w342 -> [w347 w351 w355 w364 w368 w374 w380 w386]
                            frame "Tug Off", Default {
                            }
                            frame "Manual Mode" {
                              n109 = To Word Integer(number=w352) -> (16bit integer=w348:cluster{"X":i16, "Y":i16})
                              n110 = call <vilib>:"Draw Line.vi"("picture"=w351, "end point"=w348, "color(black)"=u32 16746732, "pen"=T5 {"Width"=1, "Style"=enum."Solid"}) -> ("new picture"=w353:picture)  [unwired: 5 in]
                            }
                            frame "Back Up" {
                              n111 = To Word Integer(number=w358) -> (16bit integer=w354:cluster{"X":i16, "Y":i16})
                              n112 = call <vilib>:"Draw Line.vi"("picture"=w355, "end point"=w354, "color(black)"=u32 16719872, "pen"=T5 {"Width"=1, "Style"=enum."Dash"}) -> ("new picture"=w359:picture)  [unwired: 5 in]
                            }
                            frame "Left Wall Follow" {
                              n113 = To Word Integer(number=w361) -> (16bit integer=w362:cluster{"X":i16, "Y":i16})
                              n114 = call <vilib>:"Draw Line.vi"("picture"=w364, "end point"=w362, "color(black)"=u32 16769042, "pen"=T5 {"Width"=1, "Style"=enum."Dash"}) -> ("new picture"=w363:picture)  [unwired: 5 in]
                            }
                            frame "Goto WayPoint" {
                              n115 = To Word Integer(number=w367) -> (16bit integer=w369:cluster{"X":i16, "Y":i16})
                              n116 = call <vilib>:"Draw Line.vi"("picture"=w368, "end point"=w369, "color(black)"=u32 60927, "pen"=T5 {"Width"=1, "Style"=enum."Solid"}) -> ("new picture"=w366:picture)  [unwired: 5 in]
                            }
                            frame "Circle" {
                              n117 = To Word Integer(number=w372) -> (16bit integer=w377:cluster{"X":i16, "Y":i16})
                              n118 = call <vilib>:"Draw Line.vi"("picture"=w374, "end point"=w377, "color(black)"=u32 65351, "pen"=T5 {"Width"=1, "Style"=enum."DashDot"}) -> ("new picture"=w373:picture)  [unwired: 5 in]
                            }
                            frame "Right Wall Follow" {
                              n119 = To Word Integer(number=w378) -> (16bit integer=w383:cluster{"X":i16, "Y":i16})
                              n120 = call <vilib>:"Draw Line.vi"("picture"=w380, "end point"=w383, "color(black)"=u32 16754450, "pen"=T5 {"Width"=1, "Style"=enum."Dash"}) -> ("new picture"=w379:picture)  [unwired: 5 in]
                            }
                            frame "Hunt" {
                              n121 = To Word Integer(number=w384) -> (16bit integer=w387:cluster{"X":i16, "Y":i16})
                              n122 = call <vilib>:"Draw Line.vi"("picture"=w386, "end point"=w387, "color(black)"=u32 16720896, "pen"=T5 {"Width"=1, "Style"=enum."DashDotDot"}) -> ("new picture"=w385:picture)  [unwired: 5 in]
                            }
                          }
                        }
                      }
                      n123 = local read "initialized MDF"() -> (w338:T4)
                    }
                    event "Select Your Behavior": Value Change {
                      # "When the user selects a new operation, we disable certain controls that aren't relevant to\nthe operation that the user is performing."
                      n124 = event-data() -> ("NewVal"=w395:T7)  [unwired: 1 in]
                      n125 = property on="Select Pen Attributes" class="Clust (strict)"() -> ("Controls[]"=w394:refnum<vi>[])  [unwired: 2 in, 2 out]
                      n126 = case shown="\"Manual Mode\"" w395 {
                        tunnel: w394 -> [w399 w400 w404 w408 w412 w416 w420 w424]
                        tunnel: "Select Pen Attributes" -> [_ _ _ _ _ _ _ _]
                        frame "Manual Mode" {
                          # "All attributes are valid for this\noperation."
                          n127 = Index Array "Index Array"(array=w399, index=1) -> (element=w397:refnum<vi>)
                          n128 = property on="Property Node" class="Ctl"(reference=w397, "Disabled"=u8 0) -> ()  [unwired: 1 in, 2 out]
                        }
                        frame "Back Up" {
                          # "All attributes are valid for this\noperation."
                          n129 = Index Array(array=w400, index=1) -> (element=w402:refnum<vi>)
                          n130 = property class="Ctl"(reference=w402, "Disabled"=u8 0) -> ()  [unwired: 1 in, 2 out]
                        }
                        frame "Tug Off" {
                          # "All attributes are valid for this\noperation."
                          n131 = Index Array "Index Array"(array=w404, index=1) -> (element=w406:refnum<vi>)
                          n132 = property on="Property Node" class="Ctl"(reference=w406, "Disabled"=u8 0) -> ()  [unwired: 1 in, 2 out]
                        }
                        frame "Left Wall Follow" {
                          # "All attributes are valid for this\noperation."
                          n133 = Index Array "Index Array"(array=w408, index=1) -> (element=w410:refnum<vi>)
                          n134 = property on="Property Node" class="Ctl"(reference=w410, "Disabled"=u8 0) -> ()  [unwired: 1 in, 2 out]
                        }
                        frame "Goto WayPoint" {
                          # "All attributes are valid for this\noperation."
                          n135 = Index Array "Index Array"(array=w412, index=1) -> (element=w414:refnum<vi>)
                          n136 = property on="Property Node" class="Ctl"(reference=w414, "Disabled"=u8 0) -> ()  [unwired: 1 in, 2 out]
                        }
                        frame "Circle" {
                          # "All attributes are valid for this\noperation."
                          n137 = Index Array "Index Array"(array=w416, index=1) -> (element=w418:refnum<vi>)
                          n138 = property on="Property Node" class="Ctl"(reference=w418, "Disabled"=u8 0) -> ()  [unwired: 1 in, 2 out]
                        }
                        frame "Right Wall Follow" {
                          # "All attributes are valid for this\noperation."
                          n139 = Index Array "Index Array"(array=w420, index=1) -> (element=w422:refnum<vi>)
                          n140 = property on="Property Node" class="Ctl"(reference=w422, "Disabled"=u8 0) -> ()  [unwired: 1 in, 2 out]
                        }
                        frame "Hunt" {
                          # "All attributes are valid for this\noperation."
                          n141 = Index Array "Index Array"(array=w424, index=1) -> (element=w426:refnum<vi>)
                          n142 = property on="Property Node" class="Ctl"(reference=w426, "Disabled"=u8 0) -> ()  [unwired: 1 in, 2 out]
                        }
                      }
                      n143 = local read "initialized MDF"() -> (w392:T4)
                    }
                    event "MissionDefFile": Mouse Up {
                      # "When the user is finished drawing, we complete the operation."
                      # "Finished Drawing"
                      n144 = event-data() -> ()  [unwired: 1 in, 3 out]
                      n145 = local write "Draw??"(FALSE ("Draw??")) -> ()
                      n146 = local read "initialized MDF"() -> (w429:T4)
                    }
                  }
                  "MissionDefFile" <- w302
                  "MDF_Original" <- w300
                  n147 = call "UpdateMDF.vi"("Index"=0, "MDF_In"=w300) -> ("MDF_Out"=→"MDF":T4)  [unwired: 9 in]
                }
                n148 = Wait (ms)(milliseconds to wait=u32 200) -> ()  [unwired: 1 out]
                "Way Point Index" <- 0 ("Boundary Point Index")
              }
              frame #1 {
                w433 = T1."AutoMode" ("Tab")
                # "Force \nnext \ncase\nto  be\nAutoMode"
                n149 = local write "Tab"(w433) -> ()
                n150 = local write "Exit Planning"(FALSE ("Exit Planning")) -> ()
              }
            }
          }
          frame "ManualMode" {
            # "Removing map shift register\nfixed memory leak?"
            # "Manual Steering by dashboard heading steering wheel\nand by speed slider"
            # "This mode lets \noperator directly\ndrive robot via\nthe ManualMode\ntabbed interface"
            n151 = while {
              shift-right: [w463] -> _
              shift-left: _ -> [w462]
              tunnel: w437 -> [w455]
              shift-right: [w452] -> _
              shift-left: _ -> [w451]
              tunnel: w435 -> [w449]
              stop <- w461 stop-if-true
              # "WhereAmI?"
              n152 = Get Date/Time In Seconds "GetMiissionCurrentTime"() -> (seconds since 1Jan1904=w456:timestamp)
              n153 = call "WhereForebrainPerception.vi"("Where? Midbrain"="WhereAmI?FromBase") -> ("Where? Forebrain"=→"Where? Manual":T6, "(xr,yr)"=w452:cluster{"X":dbl, "Y":dbl}, "Direction"=w441:dbl)  [unwired: 3 in, 1 out]
              "(xr,yr)" <- w452
              n154 = local read "ManualModeStop"() -> (w461:bool)
              n155 = To Double Precision Float(number=w456) -> (double precision float=w457:dbl)
              n156 = Greater Or Equal?(x=w441, y=181.0) -> (x >= y?=w446:bool)
              n157 = local read "Manual Heading"() -> (w453:i16)
              n158 = Subtract(x=w457, y=w455) -> (x-y=w458:dbl)
              n159 = Not(x=w462) -> (.not. x?=w463:bool)
              n160 = call "DrawBuoy.vi"("(xr,yr) old"=w451, "(xr,yr) new"=w452, "2D Picture"=w449) -> ("new picture"=→"ManualMissionMap":picture)
              n161 = Divide(x=w458, y=60.0) -> (x/y=w460:dbl)
              "MissionTime" <- w460
              n162 = Subtract(x=w441, y=360.0) -> (x-y=w444:dbl)
              n163 = shared-variable "My Computer\\RobotBrainExLibrary.lvlib\\MissionTime"(w460) -> ()  [unwired: 1 in, 1 out]
              n164 = Select(t=w444, s=w446, f=w441) -> (s? t:f=w443:dbl)
              n165 = Bundle("Direction"=w443, "Manual Heading"=w453) -> (→"Heading":cluster{"Direction":dbl, "Manual Heading":i16})  [unwired: 1 in]
              n166 = Wait Until Next ms Multiple(millisecond multiple=u32 100 ("milliseconds to wait")) -> ()  [unwired: 1 out]
              "Where? 2" <- w462
            }
            n167 = while {
              shift-right: [w470] -> _
              shift-left: _ -> [w471]
              stop <- "ManualModeStop" stop-if-true
              # "WhatIsAroundMe?"
              n168 = local read "WhatAroundMeMap?"() -> (w465:cluster{"T":dbl, "Range":dbl, "Bearing":dbl}[])
              n169 = call "ProcessLidarData.vi"("WhatAroundMe?MM"=w465) -> ("Collision"=w466:bool, "data array [mag, phase (deg)]"=w467:cluster{"magnitude":dbl, "phase":dbl}[])
              "CollisionLight" <- w466
              n170 = Not(x=w471) -> (.not. x?=w470:bool)
              "MWhat?" <- w470
              n171 = call "SimLIDARPlot.vi"("data array [mag, phase (deg)]"=w467) -> ("SONAR"=→"ManualModeMapDAR":picture)  [unwired: 1 in]
              n172 = case shown="True" w466 {
                frame False {
                  # "No \nBeep"
                }
                frame True {
                  n173 = call <vilib>:"Beep.vi"("use system alert? (T)"=TRUE, "duration (msec)"=u32 1000, "frequency (Hz)"=u32 900) -> ()  [unwired: 9 in]
                }
              }
              n174 = Wait Until Next ms Multiple(millisecond multiple=u32 100 ("milliseconds to wait")) -> ()  [unwired: 1 out]
            }
            n175 = while {
              shift-right: [w494] -> _
              shift-left: _ -> [w493]
              stop <- w492 stop-if-true
              # "HowAmI?"
              n176 = local read "Battery\nVolts"() -> (w491:i16)
              n177 = local read "ManualModeStop"() -> (w492:bool)
              n178 = Not(x=w493) -> (.not. x?=w494:bool)
              n179 = Divide(x=w491, y=i16 1000) -> (x/y=→"Battery":dbl)
              n180 = Wait Until Next ms Multiple(millisecond multiple=u32 100 ("milliseconds to wait")) -> ()  [unwired: 1 out]
              "How? 2" <- w493
            }
            n181 = while {
              shift-right: [w488] -> _
              shift-left: _ -> [w487]
              stop <- w486 stop-if-true
              # "ForebrainAct"
              n182 = local read "E-Stop"() -> (w484:bool)
              n183 = local read "ManualModeStop"() -> (w486:bool)
              n184 = Select(t=0.0, s=w484, f="Manual Vel") -> (s? t:f=w481:dbl)
              n185 = To Word Integer(number=w481) -> (16bit integer=w479:i16)
              "Speed" <- w479
              n186 = local read "Send String"() -> (→"Send String to NXT":string)
              n187 = To Word Integer(number="Behavior Command") -> (16bit integer=w476:i16)
              n188 = local write "Mode"(w476) -> ()
              n189 = local write "Desired \nVelocity"(w479) -> ()
              n190 = local write "Local\nHeading"("Manual Heading") -> ()
              n191 = Not(x=w487) -> (.not. x?=w488:bool)
              n192 = Wait Until Next ms Multiple(millisecond multiple=u32 50 ("milliseconds to wait")) -> ()  [unwired: 1 out]
              "ActManual" <- w487
            }
            n193 = local read "ManualModeStop"() -> (w438:bool)
            n194 = case shown="True" w438 {
              tunnel: [TRUE ("s") w498] -> w440
              tunnel: [T1."ManualMode" ("Tab") w499] -> w439
              frame False {
              }
              frame True {
                # "Debounce tab for clean transition"
                n195 = flat-sequence {
                  tunnel: [w505] -> w499
                  tunnel: [TRUE ("s")] -> w498
                  frame #0 {
                    n196 = Wait (ms)(milliseconds to wait=u32 100) -> ()  [unwired: 1 out]
                  }
                  frame #1 {
                    w505 = T1."Startup&Shutdown" ("Tab")
                    # "Turn off\nVelocity\non \nExit"
                    n197 = local write "ManualModeStop"(FALSE ("ManualModeStop")) -> ()
                    n198 = local write "Desired \nVelocity"(i16 0 ("Desired \nVelocity")) -> ()
                    n199 = local write "Local\nHeading"(i16 0 ("Local\nHeading")) -> ()
                    n200 = local write "Mode"(i16 0 ("Mode")) -> ()
                    n201 = local write "Tab"(w505) -> ()
                  }
                }
              }
            }
          }
          frame "AutoMode" {
            n202 = flat-sequence {
              tunnel: w513 -> [_]
              tunnel: [w516] -> w511
              tunnel: w510 -> [w516]
              tunnel: w509 -> [w515]
              tunnel: [w515] -> w508
              tunnel: w507 -> [_]
              tunnel: w511 -> [w523]
              tunnel: w508 -> [w521]
              tunnel: [w598] -> w514
              tunnel: [FALSE ("s")] -> w512
              frame #0 {
                # "Run Robot\nbased on\nmission\ndefinition\nfile"
                n203 = local write "AutoMissionMap"(w515) -> ()
                n204 = while {
                  shift-right: [w519] -> _
                  shift-left: _ -> [w518]
                  stop <- "RunAutoMode" continue-if-true
                  # "Wait for Run\nbutton press\nbefore\nturning on\nAutoMode\nCode"
                  n205 = Not(x=w518) -> (.not. x?=w519:bool)
                  n206 = Wait Until Next ms Multiple(millisecond multiple=u32 100 ("milliseconds to wait")) -> ()  [unwired: 1 out]
                  "Ready" <- w518
                }
              }
              frame #1 {
                n207 = while {
                  shift-right: [w569] -> _
                  shift-left: _ -> [w560]
                  tunnel: w523 -> [w564]
                  shift-right: [w562] -> _
                  shift-left: _ -> [w563]
                  tunnel: w521 -> [w555]
                  stop <- w559 stop-if-true
                  # "WhereAmI?"
                  n208 = local read "WhereAmI?FromBase"() -> (w554:T6)
                  n209 = Get Date/Time In Seconds "GetMiissionCurrentTime"() -> (seconds since 1Jan1904=w565:timestamp)
                  n210 = call "WhereForebrainPerception.vi"("Where? Midbrain"=w554) -> ("(xr,yr)"=w562:cluster{"X":dbl, "Y":dbl}, "Direction"=w548:dbl)  [unwired: 3 in, 2 out]
                  "Robot Position" <- w562
                  n211 = local read "RunAutoMode"() -> (w559:bool)
                  n212 = Greater Or Equal?(x=w548, y=181.0) -> (x >= y?=w552:bool)
                  n213 = To Double Precision Float(number=w565) -> (double precision float=w566:dbl)
                  n214 = Subtract(x=w566, y=w564) -> (x-y=w567:dbl)
                  n215 = Not(x=w560) -> (.not. x?=w569:bool)
                  n216 = call "DrawBuoy.vi"("(xr,yr) old"=w563, "(xr,yr) new"=w562, "2D Picture"=w555) -> ("new picture"=→"AutoMissionMap":picture)
                  n217 = local read "SteerAngle"() -> (w557:dbl)
                  n218 = Divide(x=w567, y=60.0) -> (x/y=w561:dbl)
                  "MissionTimeAuto" <- w561
                  n219 = Subtract(x=w548, y=360.0) -> (x-y=w550:dbl)
                  n220 = Select(t=w550, s=w552, f=w548) -> (s? t:f=w549:dbl)
                  n221 = shared-variable "My Computer\\RobotBrainExLibrary.lvlib\\MissionTime"(w561) -> ()  [unwired: 1 in, 1 out]
                  n222 = Bundle("Direction"=w549, "SteerAngle"=w557) -> (→"A Heading":cluster{"Direction":dbl, "SteerAngle":dbl})  [unwired: 1 in]
                  n223 = Wait Until Next ms Multiple(millisecond multiple=u32 50 ("milliseconds to wait")) -> ()  [unwired: 1 out]
                  "Where?" <- w560
                }
                n224 = while {
                  shift-right: [w588] -> _
                  shift-left: _ -> [w587]
                  shift-right: [w583] -> _
                  shift-left: 0.0 ("SteerAngle") -> [w582]
                  stop <- w590 stop-if-true
                  # "needs to put out heading in local coordinates"
                  # "Think"
                  n225 = Not(x=w587) -> (.not. x?=w588:bool)
                  n226 = Or(x="Pause", y="E-Stop") -> (x .or. y?=w572:bool)
                  n227 = local read "WhereAmI?FromBase"() -> (w586:T6)
                  n228 = local read "WhatAroundMeMap?"() -> (w585:cluster{"T":dbl, "Range":dbl, "Bearing":dbl}[])
                  n229 = local read "MDF"() -> (w574:T4)
                  n230 = call "GotoWaypoint.vi"("InhibitIn"=w572, "CurrentSteerAngle"=w582, "WhatAroundMe? Clean"=w585, "WhereAmI? Clean"=w586, "MDF In"=w574) -> ("BehCom"=→"Current Behavior":T7, "MDF Out"=w577:T4, "ActCommand"=→"WayPointAct":dbl[], "Vel"=→"A Speed":dbl, "SteerAngle"=w583:dbl)  [unwired: 1 in, 1 out]
                  "SteerAngle" <- w583
                  n231 = local write "MDF"(w577) -> ()
                  n232 = local read "RunAutoMode"() -> (w590:bool)
                  n233 = local read "MDF_Original"() -> (w580:T4)
                  n234 = local read "MDF"() -> (w579:T4)
                  n235 = Select(t=w580, s="Rerun MDF", f=w579) -> (s? t:f=w576:T4)
                  n236 = local write "MDF"(w576) -> ()
                  n237 = Wait Until Next ms Multiple(millisecond multiple=u32 50 ("milliseconds to wait")) -> ()  [unwired: 1 out]
                  "Neo-C" <- w587
                }
                n238 = while {
                  shift-right: [w541] -> _
                  shift-left: _ -> [w543]
                  stop <- w540 stop-if-true
                  # "WhatIsAroundMe?"
                  n239 = local read "WhatAroundMeMap?"() -> (w537:cluster{"T":dbl, "Range":dbl, "Bearing":dbl}[])
                  n240 = call "ProcessLidarData.vi"("WhatAroundMe?MM"=w537) -> ("Collision"=w538:bool, "data array [mag, phase (deg)]"=w542:cluster{"magnitude":dbl, "phase":dbl}[])
                  "CollisionLight 2" <- w538
                  n241 = local read "RunAutoMode"() -> (w540:bool)
                  n242 = call "SimLIDARPlot.vi"("data array [mag, phase (deg)]"=w542) -> ("SONAR"=→"AutoModeLIDAR":picture)  [unwired: 1 in]
                  n243 = Not(x=w543) -> (.not. x?=w541:bool)
                  "What?" <- w541
                  n244 = case shown="True" w538 {
                    frame False {
                      # "No \nBeep"
                    }
                    frame True {
                      n245 = call <vilib>:"Beep.vi"("use system alert? (T)"=TRUE, "duration (msec)"=u32 1000, "frequency (Hz)"=u32 900) -> ()  [unwired: 9 in]
                    }
                  }
                  n246 = Wait Until Next ms Multiple(millisecond multiple=u32 50 ("milliseconds to wait")) -> ()  [unwired: 1 out]
                }
                n247 = while {
                  shift-right: [w535] -> _
                  shift-left: _ -> [w534]
                  stop <- w533 stop-if-true
                  # "HowAmI?"
                  n248 = local read "Battery\nVolts"() -> (w531:i16)
                  n249 = local read "RunAutoMode"() -> (w533:bool)
                  n250 = Not(x=w534) -> (.not. x?=w535:bool)
                  n251 = Divide(x=w531, y=i16 1000) -> (x/y=→"AutoBattery":dbl)
                  n252 = Wait Until Next ms Multiple(millisecond multiple=u32 80 ("milliseconds to wait")) -> ()  [unwired: 1 out]
                  "How?" <- w534
                }
                n253 = while {
                  shift-right: [w528] -> _
                  shift-left: _ -> [w527]
                  stop <- w526 stop-if-true
                  # "calculate desired heading.vi"
                  # "see calc desired\nheading"
                  # "convert to \noutputtin\nDesired v and\nlocal heading"
                  # "chnage arbiter to be -180 to 180"
                  # "Note:\nadd other beh to\narbiter"
                  # "ForebrainAct"
                  n254 = local read "WayPointAct"() -> (w525:dbl[])
                  n255 = local read "RunAutoMode"() -> (w526:bool)
                  n256 = Not(x=w527) -> (.not. x?=w528:bool)
                  n257 = call "ForebrainArbiter.vi"("WaypointInput"=w525) -> ("ForebrainActCom"=w524:dbl[])  [unwired: 14 in]
                  n258 = shared-variable "My Computer\\RobotBrainExLibrary.lvlib\\ActCommand"(w524) -> ()  [unwired: 1 in, 1 out]
                  n259 = Wait Until Next ms Multiple(millisecond multiple=u32 50 ("milliseconds to wait")) -> ()  [unwired: 1 out]
                  "Act" <- w527
                }
              }
              frame #2 {
                w598 = T1."Startup&Shutdown" ("Tab")
                # "Set robot Vel to 0"
                # "Reset latched run\nswitch"
                # "Force control to\nShutdown Case"
                n260 = shared-variable "My Computer\\RobotBrainExLibrary.lvlib\\ForebrainCom"(T8 {"VelCom"=0.0, "BehCom"=enum."OpenFieldTransit"} ("ForebrainCom")) -> ()  [unwired: 1 in, 1 out]
                n261 = local write "RunAutoMode"(TRUE ("RunAutoMode")) -> ()
                n262 = Initialize Array(0.0 ("element"), 90 ("dimension size")) -> (w594:dbl[])
                n263 = shared-variable "My Computer\\RobotBrainExLibrary.lvlib\\ActCommand"(w594) -> ()  [unwired: 1 in, 1 out]
                n264 = shared-variable "My Computer\\RobotBrainExLibrary.lvlib\\Xstart"(200.0 ("Xstart")) -> ()  [unwired: 1 in, 1 out]
                n265 = shared-variable "My Computer\\RobotBrainExLibrary.lvlib\\Ystart"(400.0 ("Ystart")) -> ()  [unwired: 1 in, 1 out]
                n266 = local write "Tab"(w598) -> ()
              }
            }
          }
          frame "Documentation" {
            # "Add:\n1) Blinking lights in each loop to show that they are running"
            # "This mode is just a static data flow picture of the ForeBrain"
            n267 = Wait (ms)(milliseconds to wait=u32 500) -> ()  [unwired: 1 out]
          }
          frame "DebugTHINK" {
            w608 = T1."Startup&Shutdown" ("Tab")
            # "Add:\n1) a button for each midbrain behavior to help in debugging\n2) graph of \"neural\" arbiter brain waves for each actuator\n3) a button for each forebrain behavior"
            # "Put code here in place of delay"
            # "Sends Tab Control\nback to Startup\ncase"
            n268 = Wait (ms)(milliseconds to wait=u32 5000) -> ()  [unwired: 1 out]
            n269 = local write "Tab"(w608) -> ()
          }
        }
        n270 = Not(x=w184) -> (.not. x?=w167:bool)
        "Robot Live" <- w167
      }
      n271 = while {
        tunnel: w56 -> [w80]
        tunnel: w55 -> [w79]
        tunnel: [w78] -> w53
        tunnel: [w77] -> w54
        shift-right: [w71] -> _
        shift-left: _ -> [w70]
        stop <- w81 continue-if-true
        w83 = 250  # timeout
        # "Finds and displays tugs position"
        # "runs continuously till program stops"
        # "Comminications with Base Station"
        # "receive string"
        # "If time out, post timeout and\nremove the timeout error"
        # "Read data from the port."
        n272 = Wait Until Next ms Multiple(millisecond multiple=u32 1) -> ()  [unwired: 1 out]
        n273 = UDP Read(connection ID=w80, timeout ms (25000)=w83, 8:w79) -> (data out=w72:string, error out=w84:errorcluster, 3:w77:refnum<k16>)  [unwired: 1 in, 2 out]
        n274 = local write "Base Station data rec'd"(w72) -> ()
        n275 = Unbundle By Name(w84) -> ("code"=w87:i32)
        n276 = Equal?(x=w87, y=56) -> (x = y?=w85:bool)
        "BS Time Out?" <- w85
        n277 = case shown="True" w85 {
          tunnel: [w94 errorcluster {"status"=FALSE, "code"=0, "source"=""} ("error out")] -> w78
          tunnel: w84 -> [w94 _]
          frame False {
          }
          frame True {
          }
        }
        n278 = call "PC parse the data.vi"("Nav String"=w72, "Tug"="Tug letter") -> ("Buoy locations"=w76:cluster{"regular expression":string, i32, i32}[], "Tug Location"=w74:T13, "Valid?"=w75:bool)  [unwired: 1 out]
        "Valid ?" <- w75
        n279 = local write "Buoy locations"(w76) -> ()
        n280 = case shown="True" w75 {
          tunnel: w74 -> [_ w93]
          frame False {
            # "No \nchange"
          }
          frame True {
            # "New values from BaseStation"
            n281 = shared-variable "My Computer\\RobotBrainExLibrary.lvlib\\MissionTime"() -> (w92:dbl)  [unwired: 1 in, 1 out]
            n282 = Unbundle(w93) -> (w91:i32, w90:i32, w89:i32)  [unwired: 1 out]
            n283 = local write "Tug X"(w91) -> ()
            n284 = local write "Tug Y"(w90) -> ()
            n285 = local write "Tug H"(w89) -> ()
            n286 = Bundle(w92, w91, w90, w89) -> (w88:cluster{dbl, i32, i32, i32})  [unwired: 1 in]
            n287 = local write "WhereAmI?FromBase"(w88) -> ()
          }
        }
        n288 = local read "RunRobot"() -> (w81:bool)
        n289 = Not(x=w70) -> (.not. x?=w71:bool)
        "udp rate" <- w70
      }
      n290 = while {
        tunnel: w57 -> [_]
        stop <- w125 continue-if-true
        # "loop timimng \ncontrolled externally"
        # "embed in loop to left latter"
        # "Send commands to NXT"
        n291 = local read "Desired \nVelocity"() -> (w127:i16)
        n292 = local read "Mode"() -> (w126:i16)
        n293 = local read "Local\nHeading"() -> (w128:i16)
        n294 = disable-structure shown="Disabled" {
          disable-tunnel: w128 -> [w133 w153]
          disable-tunnel: w127 -> [w132 w152]
          disable-tunnel: w126 -> [w131 _]
          disable-tunnel: [w129 w141] -> w124
          frame Disabled {
            n295 = Number To Decimal String(number=w131, width (-)=i16 2) -> (decimal integer string=w136:string)
            n296 = Number To Decimal String(number=w132, width (-)=i16 2) -> (decimal integer string=w135:string)
            n297 = Number To Decimal String(number=w133, width (-)=i16 4) -> (decimal integer string=w134:string)
            n298 = Concatenate Strings("$P", w136, w135, w134, "^") -> (w129:string)
          }
          frame Enabled {
            n299 = Build Array(u8 91 ("element"), "IR Servo", w153, w152, "# 0", "# 1", "# 2", "# 3", "# 4", "# 5", u8 93 ("element")) -> (w144:i16[])
            n300 = Add(x=w144, y=u8[] [0, 65, 65, 65, 65, 65, 65, 65, 65, 65, 0]) -> (x+y=w142:i16[])
            n301 = Byte Array To String(unsigned byte array=w142) -> (string=w141:string)
          }
        }
        n302 = local read "RunRobot"() -> (w125:bool)
        n303 = local write "Send String"(w124) -> ()
      }
      n304 = while {
        tunnel: w57 -> [_]
        stop <- w102 continue-if-true
        # "Receive information from NXT"
        n305 = local read "String Received"() -> (w107:string)
        n306 = Wait Until Next ms Multiple(millisecond multiple=u32 100) -> ()  [unwired: 1 out]
        n307 = String Subset(string=w107, offset (0)=1, length (rest)=1 ("length (rest)")) -> (substring=w106:string)
        n308 = case shown="\"N\"" w106 {
          tunnel: w107 -> [_ w109]
          frame Default {
          }
          frame "N" {
            # "0-15"
            # "Parse command \"N\""
            n309 = String Subset(string=w109, offset (0)=2, length (rest)=4 ("length (rest)")) -> (substring=w120:string)
            n310 = String Subset(string=w109, offset (0)=6, length (rest)=3 ("length (rest)")) -> (substring=w116:string)
            n311 = String Subset(string=w109, offset (0)=9, length (rest)=2 ("length (rest)")) -> (substring=w112:string)
            n312 = Decimal String To Number(string=w120) -> (number=w123:i32)  [unwired: 2 in, 1 out]
            n313 = Decimal String To Number(string=w116) -> (number=w115:i32)  [unwired: 2 in, 1 out]
            n314 = Decimal String To Number(string=w112) -> (number=w113:i32)  [unwired: 2 in, 1 out]
            n315 = To Word Integer(number=w123) -> (16bit integer=w119:i16)
            n316 = To Word Integer(number=w115) -> (16bit integer=w114:i16)
            n317 = To Long Integer(number=w113) -> (32bit integer=w108:i32)
            n318 = local write "LidarDist"(w114) -> ()
            n319 = local write "Battery\nVolts"(w119) -> ()
            n320 = local write "IR Index"(w108) -> ()
          }
        }
        n321 = local read "RunRobot"() -> (w102:bool)
      }
      n322 = while {
        stop <- w101 continue-if-true
        # "Run Simulated MapDAR"
        n323 = local read "Tug X"() -> (w99:i32)
        n324 = local read "Tug Y"() -> (w98:i32)
        n325 = local read "Tug H"() -> (w97:i32)
        n326 = Bundle "Bundle"("Tug X"=w99, "Tug Y"=w98, "Tug H"=w97) -> (w100:cluster{"Tug X":i32, "Tug Y":i32, "Tug H":i32})  [unwired: 1 in]
        n327 = call "HindbrainLIDAR_Sim.vi"("SubPosition"=w100) -> ("WhatAroundMe?"=→"WhatAroundMeMap?":cluster{"T":dbl, "Range":dbl, "Bearing":dbl}[])  [unwired: 10 in]
        n328 = local read "RunRobot"() -> (w101:bool)
      }
    }
    frame #2 {
      # "Close XBee Radio"
      # "Close UDP port"
      # "Realease LIDAR\nMemory"
      # "Reset Run \nSwitch"
      # "Shutdown Robot"
      n329 = call "Pixel_LIDAR_Close.vi"("error in (no error) 2"=w614, "Image"=w615) -> ()  [unwired: 1 in]
      n330 = local write "RunRobot"(TRUE ("RunRobot")) -> ()
      n331 = call "XB PC Close.vi"("error in (no error)"=w612, "VISA resource name"=w613) -> ()
      n332 = UDP Close(connection ID=w611, 8:w610) -> ()  [unwired: 2 out]
      "error out" <- w612
    }
  }
